vi "ADAM READ.vi"(4 "m_iDOTotal":i32, 6 "m_iDITotal":i32, 8 "error in (no error)":errorcluster caption="错误输入（无错误）", 11 "引用":refnum<k24>) -> (0 "error out":errorcluster caption="错误输出", 1 "inputresut":string[](array[string]), 2 "str_DI":string[](array[string]), 3 "str_DO":string[](array[string]), 5 "引用输出":refnum<k24>)   [LabVIEW 2017]
uses:
  ADAM-4050DLL.dll
panel:
  in  "input":bool[](array[boolean])=[FALSE, FALSE, FALSE, FALSE, FALSE, FALSE, FALSE, FALSE]
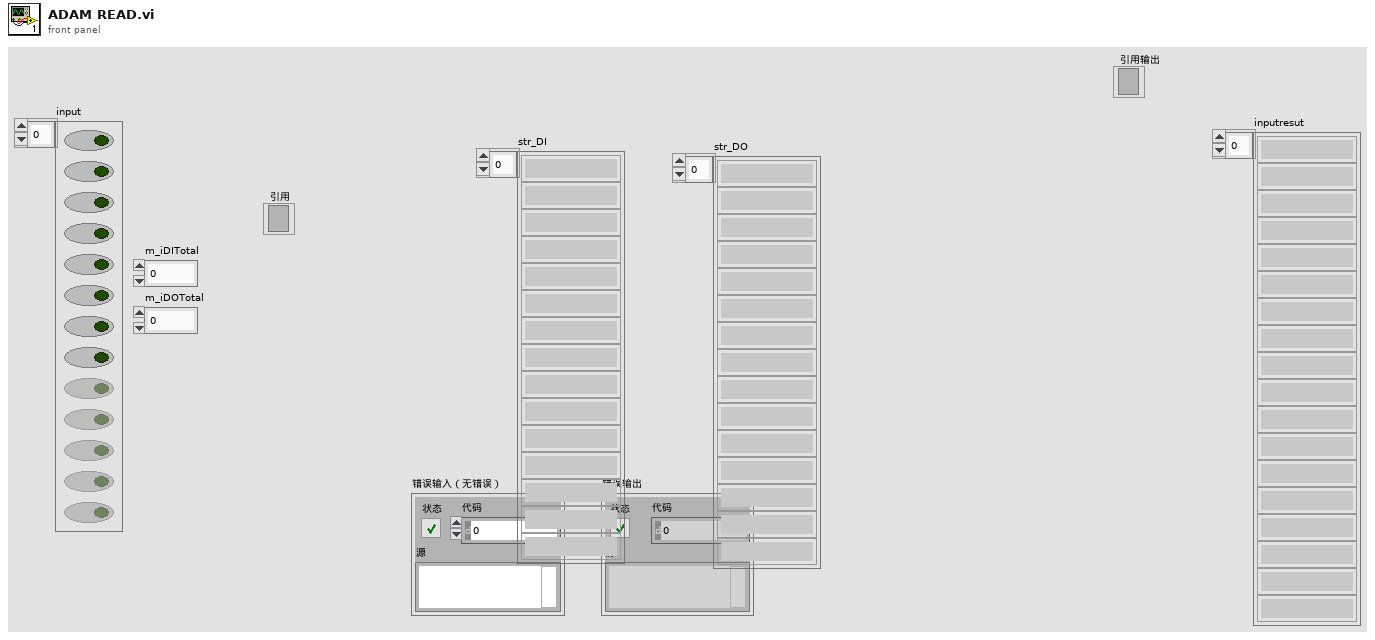
[diagram p1: front panel]
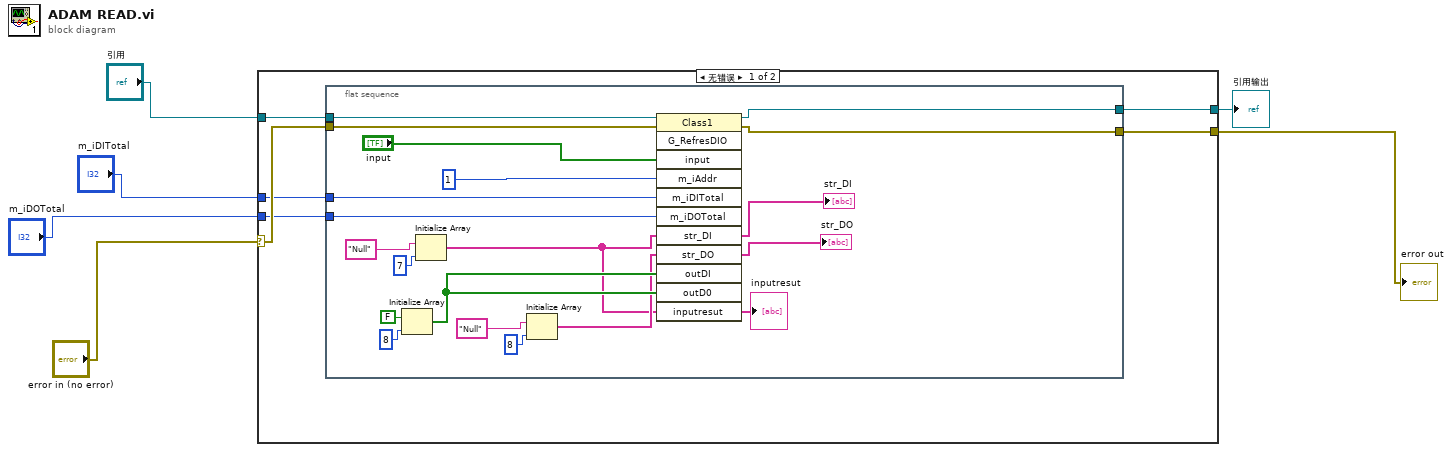
[diagram p0: block diagram]
diagram:
  n1 = case shown="无错误" "error in (no error)" {
    selector: "error in (no error)" -> [w11 _]
    tunnel: [w12 _] -> w6
    tunnel: "m_iDITotal" -> [w10 _]
    tunnel: "m_iDOTotal" -> [w9 _]
    tunnel: "引用" -> [w8 _]
    tunnel: [w7 _] -> w1
    frame No Error {
      n2 = flat-sequence {
        tunnel: [w32] -> w12
        tunnel: w11 -> [w17]
        tunnel: w10 -> [w16]
        tunnel: w9 -> [w15]
        tunnel: w8 -> [w14]
        tunnel: [w13] -> w7
        frame #0 {
          n3 = Initialize Array(FALSE, 8 ("维数大小")) -> (w27:bool[])
          n4 = Initialize Array("Null", 7 ("维数大小")) -> (w20:string[])
          n5 = Initialize Array("Null", 8 ("维数大小")) -> (w21:string[])
          n6 = invoke class="Class1" method="G_RefresDIO"(reference=w14, error in=w17, "input"="input", "m_iAddr"=1, "m_iDITotal"=w16, "m_iDOTotal"=w15, "str_DI"=w20, "str_DO"=w21, "outDI"=w27, "outD0"=w27, "inputresut"=w20) -> (reference out=w13:refnum<k24>, error out=w32:errorcluster, "str_DI"=→"str_DI":string[], "str_DO"=→"str_DO":string[], "inputresut"=→"inputresut":string[])  [unwired: 1 in, 7 out]
        }
      }
    }
    frame Error {
    }
  }
  "error out" <- w6
  "引用输出" <- w1
